vi "CE Load XCL template.vi"(8 "error in (no error)":errorcluster, 11 "CE measurement":T1={"Signal frequencies (Hz) T"=[1000.0], "Signal amplitudes (V) T"=[0.707], "Sampling frequencies (Hz) T"=[10000000.0], "Record lengths (multiples of periods) T"=[10000.0], "TWM data root directory"=path "", "TWM mreasurements directories"=[], "Calculate RMS from samples"=FALSE, "Algorithm to use"="TWM-WFFT", "Quantity to read"="TWM-WFFT", "Settle down after AC source change (s) T"=1.0, "Skip PJVS setup"=FALSE, "Measurement template file"=path "", "Row of START keyword T"=0, "Row of STOP keyword T"=0, "Measurement template line T"=[], "Switch position T"=[10000.0], "FR fit mat file T"=path "", "Recalculate-skip already calculated"=FALSE} {"Switch position T" format="%#_3p"; "Record lengths (multiples of periods) T" format="%#_3p"; "Sampling frequencies (Hz) T" format="%#_3p"; "Signal amplitudes (V) T" format="%#_3p"; "Signal frequencies (Hz) T" format="%#_3p"}) -> (0 "error out":errorcluster, 3 "CE measurement out":T1={"Signal frequencies (Hz) T"=[1000.0], "Signal amplitudes (V) T"=[0.707], "Sampling frequencies (Hz) T"=[10000000.0], "Record lengths (multiples of periods) T"=[10000.0], "TWM data root directory"=path "", "TWM mreasurements directories"=[], "Calculate RMS from samples"=FALSE, "Algorithm to use"="TWM-WFFT", "Quantity to read"="TWM-WFFT", "Settle down after AC source change (s) T"=1.0, "Skip PJVS setup"=FALSE, "Measurement template file"=path "", "Row of START keyword T"=0, "Row of STOP keyword T"=0, "Measurement template line T"=[], "Switch position T"=[10000.0], "FR fit mat file T"=path "", "Recalculate-skip already calculated"=FALSE} {"Switch position T" format="%#_3p"; "Record lengths (multiples of periods) T" format="%#_3p"; "Sampling frequencies (Hz) T" format="%#_3p"; "Signal amplitudes (V) T" format="%#_3p"; "Signal frequencies (Hz) T" format="%#_3p"})   [LabVIEW 2020]
doc: "Reads values from CE measurement template in excell spreadsheet."
uses:
  CE Measurement/Type definitions/CE measurement.ctl
  <vilib>/Utility/NIReport.llb/Report Type.ctl
  <vilib>/Utility/error.llb/DialogType.ctl
  <vilib>/addons/_office/excel.llb/Excel Get Data ([str]).vi
  <vilib>/Utility/NIReport.llb/NI_report.lvclass
  <vilib>/addons/_office/NI_ReportGenerationToolkit.lvlib
  <vilib>/Utility/NIReport.llb/NI_ReportGenerationCore.lvlib
  <vilib>/Utility/NIReport.llb/Excel/NI_Excel.lvclass
panel:
  out "Stop row":i32
  out "Start row":i32
  out "excell template content":string[][](array[string])
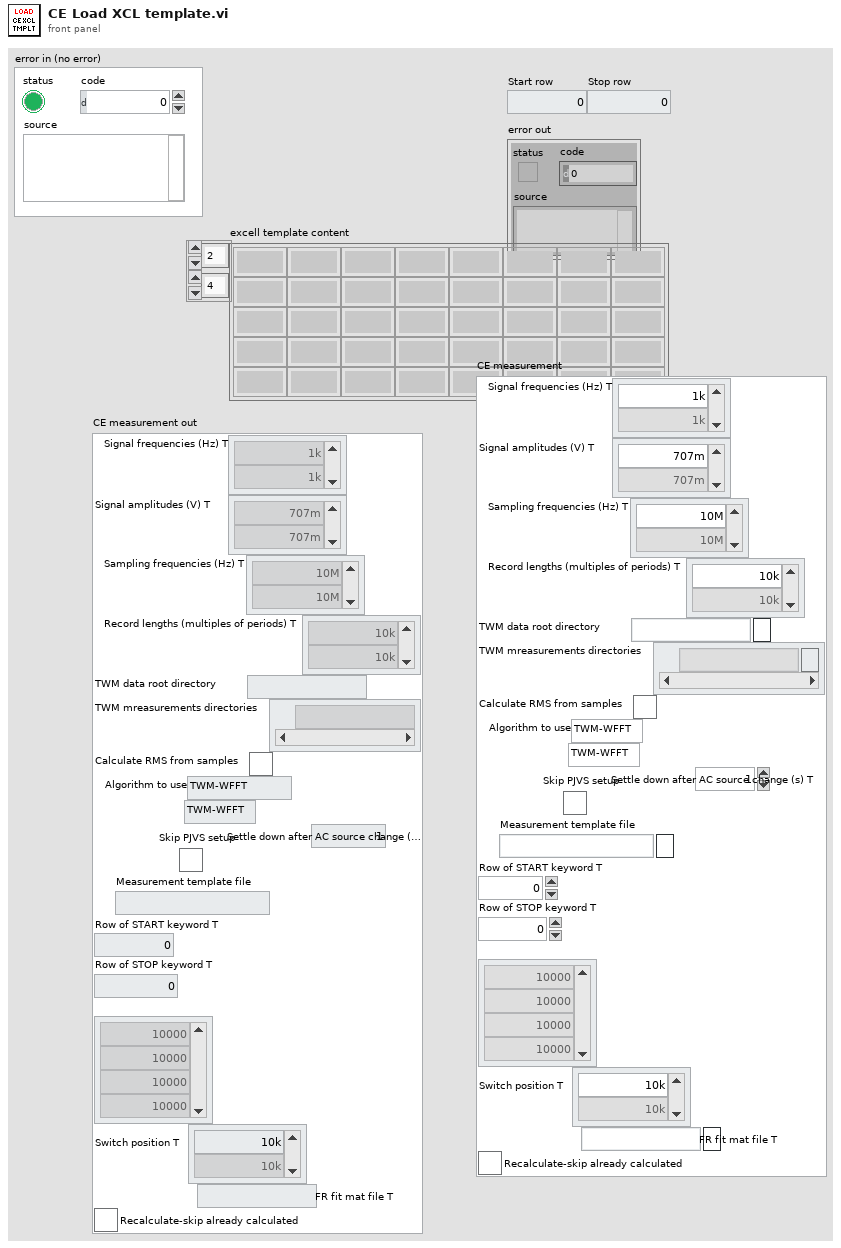
[diagram p1: front panel]
types:
  T1 = typedef "CE measurement.ctl" = cluster{"Signal frequencies (Hz) T":dbl[], "Signal amplitudes (V) T":dbl[], "Sampling frequencies (Hz) T":dbl[], "Record lengths (multiples of periods) T":dbl[], "TWM data root directory":path, "TWM mreasurements directories":path[], "Calculate RMS from samples":bool, "Algorithm to use":string, "Quantity to read":string, "Settle down after AC source change (s) T":dbl, "Skip PJVS setup":bool, "Measurement template file":path, "Row of START keyword T":i32, "Row of STOP keyword T":i32, "Measurement template line T":i32[], "Switch position T":dbl[], "FR fit mat file T":path, "Recalculate-skip already calculated":bool}
  T2 = enum16{"maximized", "minimized", "normal", "no change"}
  T3 = typedef "NI_ReportGenerationCore.lvlib/Report Type.ctl" = enum16{"HTML", "Word", "Excel"}
  T4 = typedef "Type definitions to be saved.ctl" = cluster{"Common properties":T5, "AC Source":T6, "DC meter":T8, "CE measurement":T1, "FR measurement":T10, "FR template":T11, "CE template":T12, "PJVS":T13, "SS measurement":T17, "AC sync source":T6, "DG measurement":T18}
  T5 = typedef "Common properties.ctl" = cluster{"Measurement status ref":refnum<vi>, "TWM Status ref":refnum<vi>, "Abort ref":refnum<vi>, "Skip waiting ref":refnum<vi>, "GNU Octave path":path, "TWM+QWTB path":path, "lvlib path":path, "TWM pipe":string, "PJVS status ref":refnum<vi>, "WAC path":path}
  T6 = typedef "AC Source.ctl" = cluster{"AC Source type":T7, "VISA":refnum<visa-resource-name>, "Ref. clock (Hz)":dbl, "status ref":refnum<vi>, "Fluke 57XX wideband output":bool, "Fluke 57XX ignore errors":bool, "Synchronization by AC signal":bool}
  T7 = typedef "AC Source type.ctl" = enum16{"Fluke 5XXX calibrator", "Tektronix AFG3000 series", "dummy", "Agilent 331xxA to 332xxA", "Agilent 335xxA to 336xxA"}
  T8 = typedef "DC meter.ctl" = cluster{"DC meter type":T9, "DC meter VISA":refnum<visa-resource-name>, "NPLC":dbl, "status ref":refnum<vi>}
  T9 = typedef "DC meter type.ctl" = enum16{"H/A/K 3458", "Fluke 8508A", "dummy", "Keithley 2182"}
  T10 = typedef "FR measuement.ctl" = cluster{"Measurement frequencies (Hz)":dbl[], "Sampling frequency (Hz)":dbl, "Signal amplitude (V)":dbl, "AC-DC settle time (s)":dbl, "Record length (multiples of period)":dbl[], "Measurement template file":path, "Row of START keyword":i32, "Row of STOP keyword":i32, "Calculate RMS from samples":bool, "AC-DC warm up time (s)":dbl, "Measurement template line":i32[], "DC meter readings No.":i32, "Algorithm":string, "Simultaneous measurement":bool, "Recalculate-skip already calculated":bool}
  T11 = typedef "FR template.ctl" = cluster{"Keywords column":i32, "Sig. freq. column":i32, "Rec. len. column":i32, "Meas. points. row min to read":i32, "Meas. points. row max to read":i32, "Properties column":i32, "Properties row start":i32, "Properties row end":i32, "Keyword START regexp":string, "Keyword STOP regexp":string, "HW data column":i32, "HW data row start":i32, "HW data row end":i32, "TIme and date column start":i32, "Digitizer value column start ":i32, "DC mean column start ":i32, "DC readings column start":i32}
  T12 = typedef "CE template.ctl" = cluster{"Keywords column":i32, "Sig. freq. column":i32, "Rec. len. column":i32, "Switch pos column":i32, "Meas. points. row min to read":i32, "Meas. points. row max to read":i32, "Properties column":i32, "Properties row start":i32, "Properties row end":i32, "Keyword START regexp":string, "Keyword STOP regexp":string, "HW data column":i32, "HW data row start":i32, "HW data row end":i32, "TIme and date column start":i32, "Digitizer value column start ":i32}
  T13 = typedef "PJVS.ctl" = cluster{"PJVS type":T14, "Status Refnum":refnum<vi>, "AC-supraVOLTcontrol":cluster{"IP address:port (0.0.0.0:0000)":string, "Timeouts":T15, "Simulation mode":bool, "Debug mode":bool}, "NPL bias source":cluster{"DataSocketCluster":T16}, "Manual PJVS":cluster{"PJVS frequency (Hz)":dbl, "Reference voltages (V)":dbl[], "File with PJVS voltages":path}, "VTT PJVS":cluster{"some VTT only property":string}}
  T14 = typedef "PJVS Type.ctl" = enum16{"AC-supraVOLTcontrol", "JV modified NPL bias control", "Manual PJVS", "VTT PJVS"}
  T15 = typedef "ACSVcontrol-driver.lvlib/Timeouts.ctl" = cluster{"TCP Read & Write (ms)":i32, "Sensors readout":i32, "PJVS setup":i32, "Nullmeter readout":i32, "Multiplexer setup":i32, "57XX setup":i32, "Generator setup":i32, "Synthesizer setup":i32, "Sampler readout":i32}
  T16 = typedef "DataSocketCluster external.ctl" = cluster{"Server Machine":string, "Client Machine":string, "Data":string, "TimeStamp":dbl, "Count":i32, "Target Process":string}
  T17 = typedef "SS measurement.ctl" = cluster{"Signal frequencies (Hz)":dbl[], "Signal amplitudes (V)":dbl[], "Sampling frequencies (Hz)":dbl[], "Record lengths (multiples of periods)":dbl[], "Calculate results":bool, "Algorithm":string, "TWM data directories":path[], "TWM data directories relative":path[], "Settle down after AC source change (s)":dbl, "PJVS frequencies (Hz)":dbl[], "PJVS reference voltages array of vector cluster":cluster{"PJVS reference voltages vector":dbl[]}[], "Requested PJVS steps":u32[], "Measure CE":bool, "Measure CE before":bool, "Measure CE after":bool, "Single point CE measurement":bool, "original CE template path":path, "new CE template path before SS":path, "new CE template path before SS relative":path, "new CE template path after SS":path, "new CE template path after SS relative":path, "original CE fit path":path, "new CE fit path before SS":path, "new CE fit path before SS relative":path, "new CE fit path after SS":path, "new CE fit path after SS relative":path, "Measure digitizer gain":bool, "Measure digitizer gain before":bool, "Measure digitizer gain after":bool, "Digitizer gain":dbl, "Data folder":path, "FR fit path":path, "new FR fit path relative":path, "Rs":i32, "Re":i32, "SS measurement info files":path[]}
  T18 = typedef "DG measurement.ctl" = cluster{"Sampling frequencies (Hz)":dbl[], "Requested PJVS frequencies (Hz)":dbl[], "Requested PJVS waveform amplitudes (V)":dbl[], "Record lengths (multiples of PJVS periods)":dbl[], "Requested PJVS steps":u32[], "Switch position":dbl, "Settle down after PJVS change (s)":dbl, "Rs":i32, "Re":i32, "Algorithm":string, "Calculate results":bool, "Data folder":path, "TWM data directories":path[], "TWM data directories relative":path[], "DG measurement info files":path[], "Set PJVS frequencies (Hz)":dbl[], "Set PJVS reference voltages array of vector cluster":cluster{"PJVS reference voltages vector":dbl[]}[], "Set PJVS steps":u32[]}
  T19 = typedef "DialogType.ctl" = u16
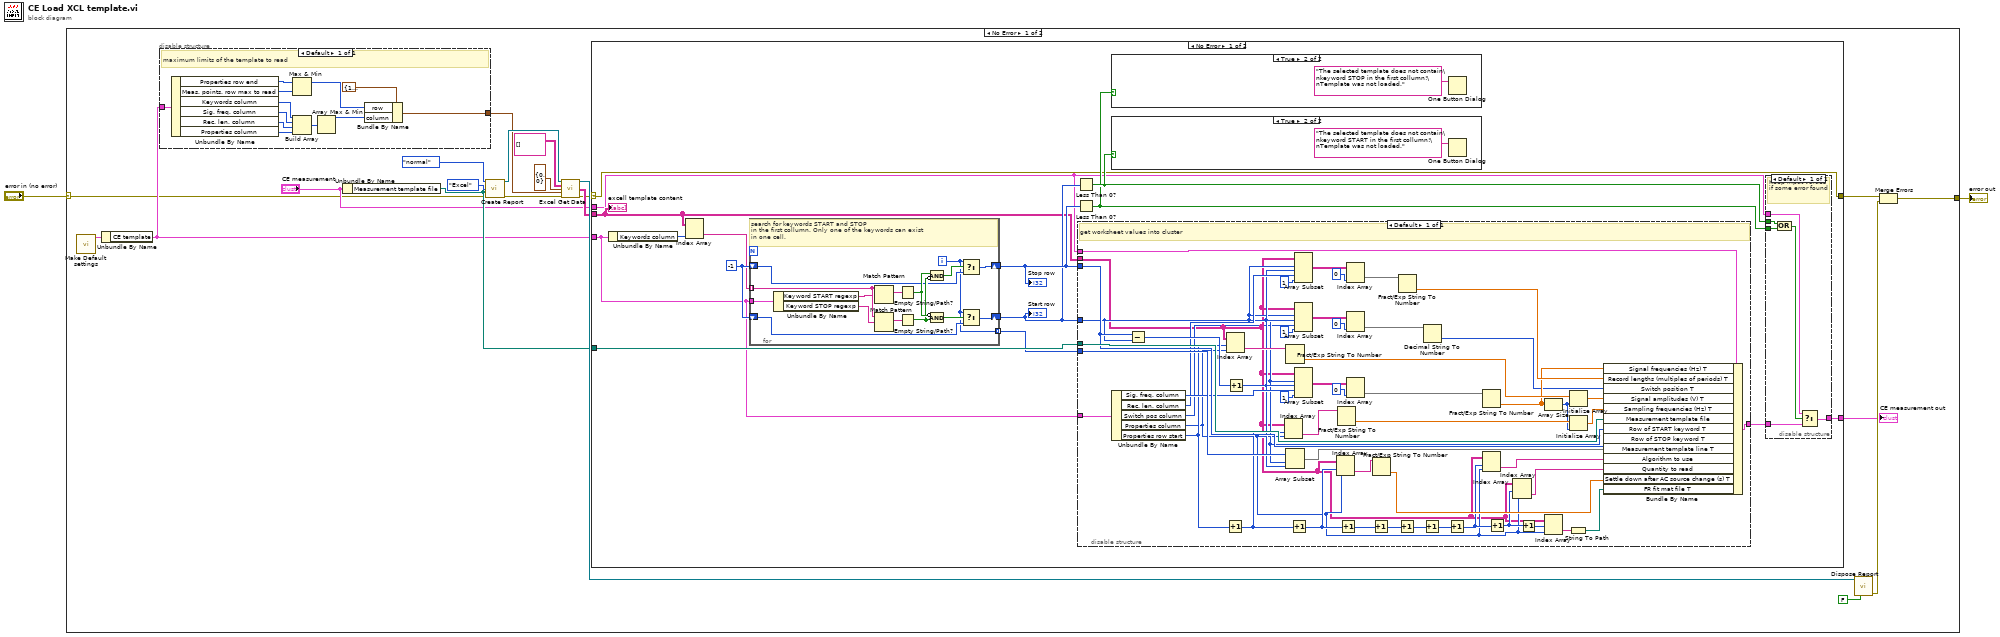
[diagram p0: block diagram]
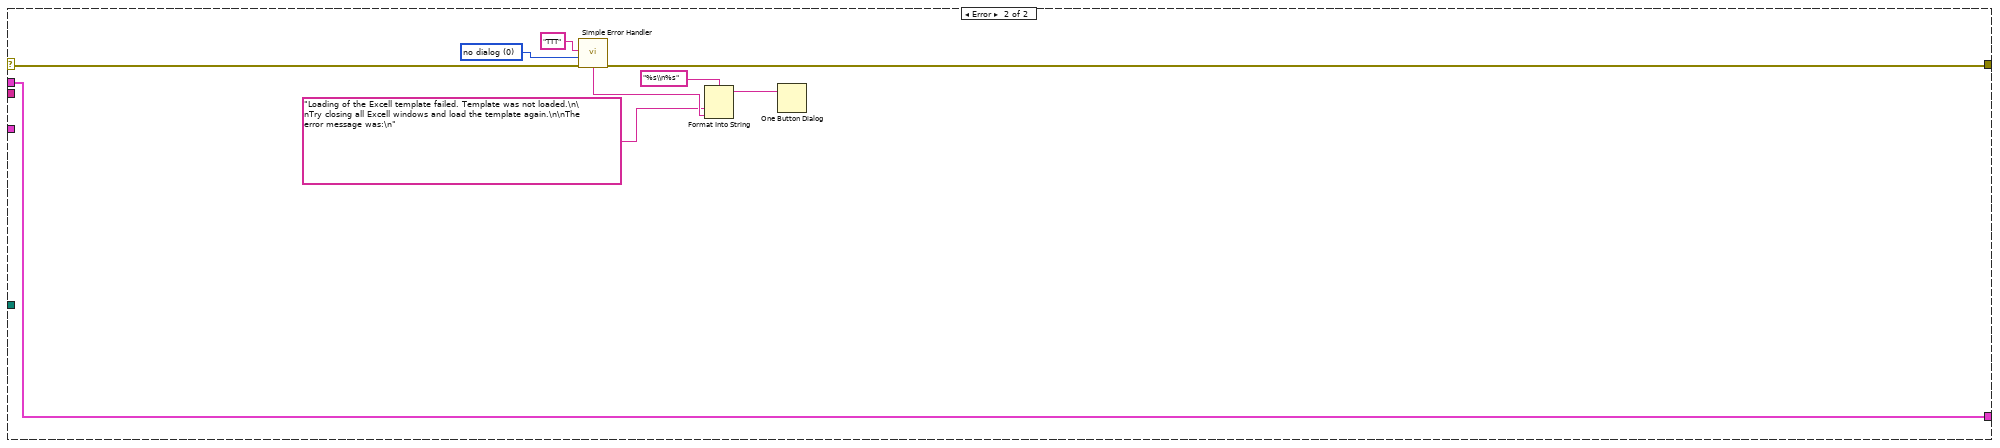
[diagram p4: hidden frame]
diagram:
  n1 = case shown="No Error" "error in (no error)" {
    selector: "error in (no error)" -> [w3 w135]
    tunnel: [w4 w135] -> w2
    frame No Error {
      n2 = call "Make Default settings.vi"() -> ("TD to be saved"=w9:T4)  [unwired: 11 in]
      n3 = Unbundle By Name(w9) -> ("CE template"=w7:T12)
      n4 = disable-structure shown="Default" {
        disable-tunnel: w7 -> [w34]
        disable-tunnel: [w32] -> w10
        frame Enabled {
          # "maximum limits of the template to read"
          n5 = Unbundle By Name(w34) -> ("Properties row end"=w25:i32, "Meas. points. row max to read"=w24:i32, "Keywords column"=w31:i32, "Sig. freq. column"=w30:i32, "Rec. len. column"=w29:i32, "Properties column"=w28:i32)
          n6 = Max & Min(x=w25, y=w24) -> (max(x,y)=w23:i32)  [unwired: 1 out]
          n7 = Build Array(w31, w30, w29, w28) -> (w27:i32[])
          n8 = Array Max & Min(array=w27) -> (max value=w26:i32)  [unwired: 3 out]
          n9 = Bundle By Name(cluster=cluster{"row":i32, "column":i32} {"row"=100000, "column"=7} ("end (-1, -1)"), "row"=w23, "column"=w26) -> (w32:cluster{"row":i32, "column":i32})
        }
      }
      n10 = Unbundle By Name("CE measurement") -> ("Measurement template file"=w8:path)
      n11 = call <vilib>:"Create Report.vi"("window state (normal)"=T2."normal", "report type"=Report_Type."Excel", "template (empty)"=w8, "error in (no error)"=w3) -> ("report out"=w22:refnum<class "NI_report.lvclass">, "error out"=w21:errorcluster)  [unwired: 10 in]
      n12 = call-poly <vilib>:"Excel Get Data.vi"("report in"=w22, "data type"=string[][] [], "start (-1, -1)"=cluster{"row":i32, "column":i32} {"row"=0, "column"=0}, "end (-1, -1)"=w10, "error in (no error)"=w21) -> ("report out"=w20:refnum<class "NI_report.lvclass">, "data"=w16:string[][], "error out"=w13:errorcluster)  [unwired: 8 in]
      n13 = case shown="No Error" w13 {
        selector: w13 -> [w38 w133]
        tunnel: w16 -> [w45 _]
        tunnel: [w41 w134] -> w5
        tunnel: "CE measurement" -> [w40 w134]
        tunnel: w8 -> [w39 _]
        tunnel: [w38 w130] -> w12
        tunnel: w7 -> [w36 _]
        frame No Error {
          w49 = -1
          n14 = Unbundle By Name(w36) -> ("Keywords column"=w35:i32)
          n15 = Index Array(array=w45, index (col)=w35) -> (element=w48:string[])  [unwired: 1 in]
          n16 = for {
            tunnel: w48 -> [w125] mode=indexing
            shift-right: [w121] -> w46
            shift-left: w49 -> [w115]
            shift-right: [w117] -> w47
            shift-left: w49 -> [w116]
            tunnel: [w114] -> w37 mode=indexing
            tunnel: w36 -> [w113]
            i -> [w114]
            # "search for keywords START and STOP\nin the first collumn. Only one of the keywords can exist\nin one cell."
            n17 = Unbundle By Name(w113) -> ("Keyword START regexp"=w112:string, "Keyword STOP regexp"=w111:string)
            n18 = Match Pattern(string=w125, regular expression=w112) -> (match substring=w124:string)  [unwired: 1 in, 3 out]
            n19 = Match Pattern(string=w125, regular expression=w111) -> (match substring=w123:string)  [unwired: 1 in, 3 out]
            n20 = Empty String/Path?(string/path=w124) -> (empty?=w120:bool)
            n21 = Empty String/Path?(string/path=w123) -> (empty?=w119:bool)
            n22 = Compound Arithmetic op=AND(w120, invert w119) -> (w118:bool)
            n23 = Compound Arithmetic op=AND(invert w120, w119) -> (w122:bool)
            n24 = Select(t=w114, s=w118, f=w116) -> (s? t:f=w117:i32)
            n25 = Select(t=w114, s=w122, f=w115) -> (s? t:f=w121:i32)
          }
          "Start row" <- w46
          "Stop row" <- w47
          n26 = Less Than 0?(x=w46) -> (x < 0?=w44:bool)
          n27 = Less Than 0?(x=w47) -> (x < 0?=w43:bool)
          n28 = disable-structure shown="Default" {
            disable-tunnel: w47 -> [w94]
            disable-tunnel: w46 -> [w78]
            disable-tunnel: w40 -> [w108]
            disable-tunnel: w45 -> [w57]
            disable-tunnel: [w103] -> w42
            disable-tunnel: w39 -> [w95]
            disable-tunnel: w37 -> [w93]
            disable-tunnel: w36 -> [w90]
            frame Enabled {
              # "get worksheet values into cluster"
              n29 = Unbundle By Name(w90) -> ("Sig. freq. column"=w89:i32, "Rec. len. column"=w88:i32, "Switch pos column"=w77:i32, "Properties column"=w58:i32, "Properties row start"=w87:i32)
              n30 = Subtract(x=w94, y=w78) -> (x-y=w92:i32)
              n31 = Index Array(array=w57, index (row)=w87, index (col)=w58) -> (element=w97:string)
              n32 = Increment(x=w87) -> (x+1=w70:i32)
              n33 = Increment(x=w92) -> (x+1=w79:i32)
              n34 = Index Array(array=w57, index (row)=w70, index (col)=w58) -> (element=w96:string)
              n35 = Fract/Exp String To Number(string=w97) -> (number=w86:dbl)  [unwired: 3 in, 1 out]
              n36 = Array Subset(array=w93, index=w78, length=w79) -> (w91:i32[])
              n37 = Increment(x=w70) -> (x+1=w68:i32)
              n38 = Array Subset(array=w57, index (row)=w78, length (row)=w79, index (col)=w88, length (col)=1 ("length")) -> (w100:string[][])
              n39 = Array Subset(array=w57, index (row)=w78, length (row)=w79, index (col)=w77, length (col)=1 ("length")) -> (w75:string[][])
              n40 = Array Subset(array=w57, index (row)=w78, length (row)=w79, index (col)=w89, length (col)=1 ("length")) -> (w106:string[][])
              n41 = Index Array(array=w57, index (row)=w68, index (col)=w58) -> (element=w71:string)
              n42 = Fract/Exp String To Number(string=w96) -> (number=w83:dbl)  [unwired: 3 in, 1 out]
              n43 = Increment(x=w68) -> (x+1=w67:i32)
              n44 = Index Array(array=w100, index (col)=0 ("index (row)")) -> (element=w102:string[])  [unwired: 1 in]
              n45 = Index Array(array=w75, index (col)=0 ("index (row)")) -> (element=w74:string[])  [unwired: 1 in]
              n46 = Index Array(array=w106, index (col)=0 ("index (row)")) -> (element=w104:string[])  [unwired: 1 in]
              n47 = Increment(x=w67) -> (x+1=w66:i32)
              n48 = Fract/Exp String To Number(string=w71) -> (number=w61:dbl)  [unwired: 3 in, 1 out]
              n49 = Increment(x=w66) -> (x+1=w63:i32)
              n50 = Fract/Exp String To Number(string=w102) -> (number=w98:dbl[])  [unwired: 3 in, 1 out]
              n51 = Increment(x=w63) -> (x+1=w62:i32)
              n52 = Decimal String To Number(string=w74) -> (number=w73:i32[])  [unwired: 2 in, 1 out]
              n53 = Increment(x=w62) -> (x+1=w60:i32)
              n54 = Fract/Exp String To Number(string=w104) -> (number=w85:dbl[])  [unwired: 3 in, 1 out]
              n55 = Index Array(array=w57, index (row)=w60, index (col)=w58) -> (element=w72:string)
              n56 = Increment(x=w60) -> (x+1=w59:i32)
              n57 = Index Array(array=w57, index (row)=w59, index (col)=w58) -> (element=w56:string)
              n58 = Increment(x=w59) -> (x+1=w64:i32)
              n59 = Array Size(array=w85) -> (size(s)=w82:i32)
              n60 = Index Array(array=w57, index (row)=w64, index (col)=w58) -> (element=w69:string)
              n61 = String To Path(string=w69) -> (path=w65:path)
              n62 = Initialize Array(w86, w82) -> (w84:dbl[])
              n63 = Initialize Array(w83, w82) -> (w81:dbl[])
              n64 = Bundle By Name(cluster=w108, "Signal frequencies (Hz) T"=w85, "Record lengths (multiples of periods) T"=w98, "Switch position T"=w73, "Signal amplitudes (V) T"=w84, "Sampling frequencies (Hz) T"=w81, "Measurement template file"=w95, "Row of START keyword T"=w78, "Row of STOP keyword T"=w94, "Measurement template line T"=w91, "Algorithm to use"=w72, "Quantity to read"=w56, "Settle down after AC source change (s) T"=w61, "FR fit mat file T"=w65) -> (w103:T1)
            }
          }
          n65 = case shown="True" w43 {
            frame False {
            }
            frame True {
              n66 = One Button Dialog(message="The selected template does not contain\nkeyword STOP in the first collumn!\nTemplate was not loaded.") -> ()  [unwired: 1 in, 1 out]
            }
          }
          n67 = case shown="True" w44 {
            frame False {
            }
            frame True {
              n68 = One Button Dialog(message="The selected template does not contain\nkeyword START in the first collumn!\nTemplate was not loaded.") -> ()  [unwired: 1 in, 1 out]
            }
          }
          n69 = disable-structure shown="Default" {
            disable-tunnel: w44 -> [w54]
            disable-tunnel: w43 -> [w53]
            disable-tunnel: w42 -> [w52]
            disable-tunnel: [w51] -> w41
            disable-tunnel: w40 -> [w50]
            frame Enabled {
              # "Keep input values\nif some error found"
              n70 = Compound Arithmetic op=OR(w54, w53) -> (w55:bool)
              n71 = Select(t=w50, s=w55, f=w52) -> (s? t:f=w51:T1)
            }
          }
          "excell template content" <- w45
        }
        frame Error {
          w132 = T19 0 items=["no dialog", "OK message", "continue or stop message", "OK message + warnings", "continue/stop + warnings"] ("type of dialog (OK msg:1)")
          n72 = call <vilib>:"Simple Error Handler.vi"("error source (\" \")"="TTT" ("error source (\" \")"), "type of dialog (OK msg:1)"=w132, "error in (no error)"=w133) -> ("error out"=w130:errorcluster, "message"=w127:string)  [unwired: 2 in, 3 out]
          n73 = Format Into String(format string="%s\\n%s", "Loading of the Excell template failed. Template was not loaded.\n\nTry closing all Excell windows and load the template again.\n\nThe error message was:\n" ("input 1"), w127) -> (resulting string=w128:string)  [unwired: 2 in, 1 out]
          n74 = One Button Dialog(message=w128) -> ()  [unwired: 1 in, 1 out]
        }
      }
      "CE measurement out" <- w5
      n75 = call-dynamic "Dispose Report.vi"("report in"=w20, "close report? (T)"=FALSE) -> ("error out"=w11:errorcluster)  [unwired: 13 in]
      n76 = Merge Errors(w12, w11) -> (w4:errorcluster)
    }
    frame Error {
    }
  }
  "error out" <- w2
